vi "sensor test.vi"() -> ()   [LabVIEW 2019]
uses:
  <vilib>/vision/NI_Vision_Development_Module.lvlib
  defectsWrapper/defectsWrapper.lvlib
panel:
  out "sensor errors 2":errorcluster
  in  "stop 4":bool
  out "counter out":dbl
  out "defnum":dbl
  out "proc. ok":bool=TRUE
  out "x-y defects locs":dbl[][](array[numeric])
  in  "stop 3":bool
  out "crop array":dbl[][](array[numeric])
  out "Frm False":bool
  out "Pallet Defects View":T1(plugin-control)
  in  "size":dbl=5.0
  in  "threshoulds":dbl[](array[numeric])=[900.0, 1000.0, 1600.0, 2400.0, 3000.0, 3000.0]
  out "pallet detect":bool
  out "column count":bool
  out "error out 2":errorcluster
  in  "File Path":path=path "C:/Users/user/Pictures/saved pic"
  out "error out":errorcluster
  out "speed":dbl
  out "Image":T1(plugin-control)
  in  "stop 2":bool
  out "Image Out":T1(plugin-control)
  in  "Stop (F)":bool
  out "Waveform Chart 3":waveform(dbl)(graph)
  in  "Graph Button":bool
  out "capture or not?":bool=TRUE
  in  "capture":bool
  out "capture triger":bool
  in  "Color Box 4":u32(colorbox)=16448250
  in  "counting role":T2(ring)
  in  "timout":u32=50
  in  "Remote Port":u16=502
  out "IP #":string="169.254.116.245"
  in  "3rd sensor thr":u16=50000
  in  "2nd sensor thr":u16=52000
  in  "1st sensor thr":u32=52000
  in  "stop":bool
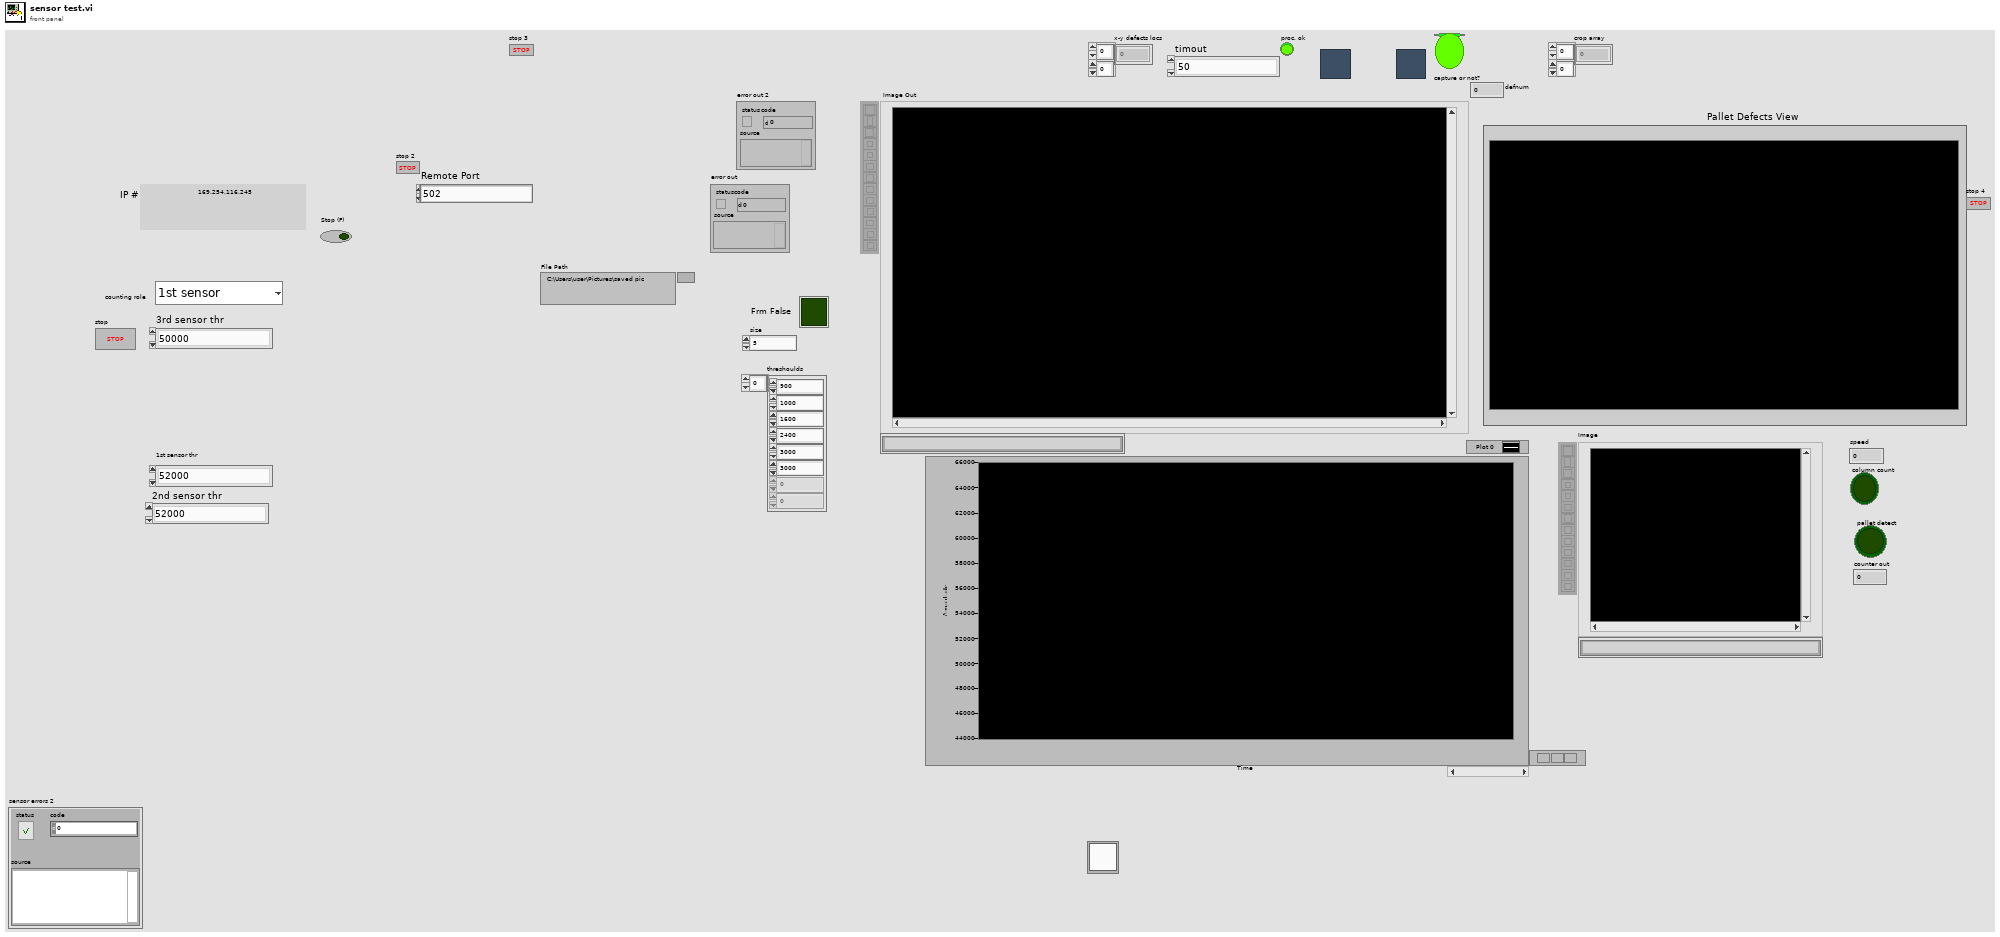
[diagram p1: front panel]
types:
  T1 = typedef "IMAQ Image.ctl" = refnum<image>
  T2 = enum16{"1st sensor", "2nd sensor", "3rd sensor", "1st+2nd", "1st+3rd", "2nd+3rd", "1st+2nd+3rd"}
  T3 = cluster{"ch sensor1":dbl, "ch sensor2":dbl, "ch sensor3":dbl, "ch sw sensor1":dbl, "ch sw sensor2":dbl}
  T4 = typedef "Image Type" = u32
  T5 = enum32{"Invalid", "Standard", "Closed", "Hidden", "Minimized", "Maximized"}
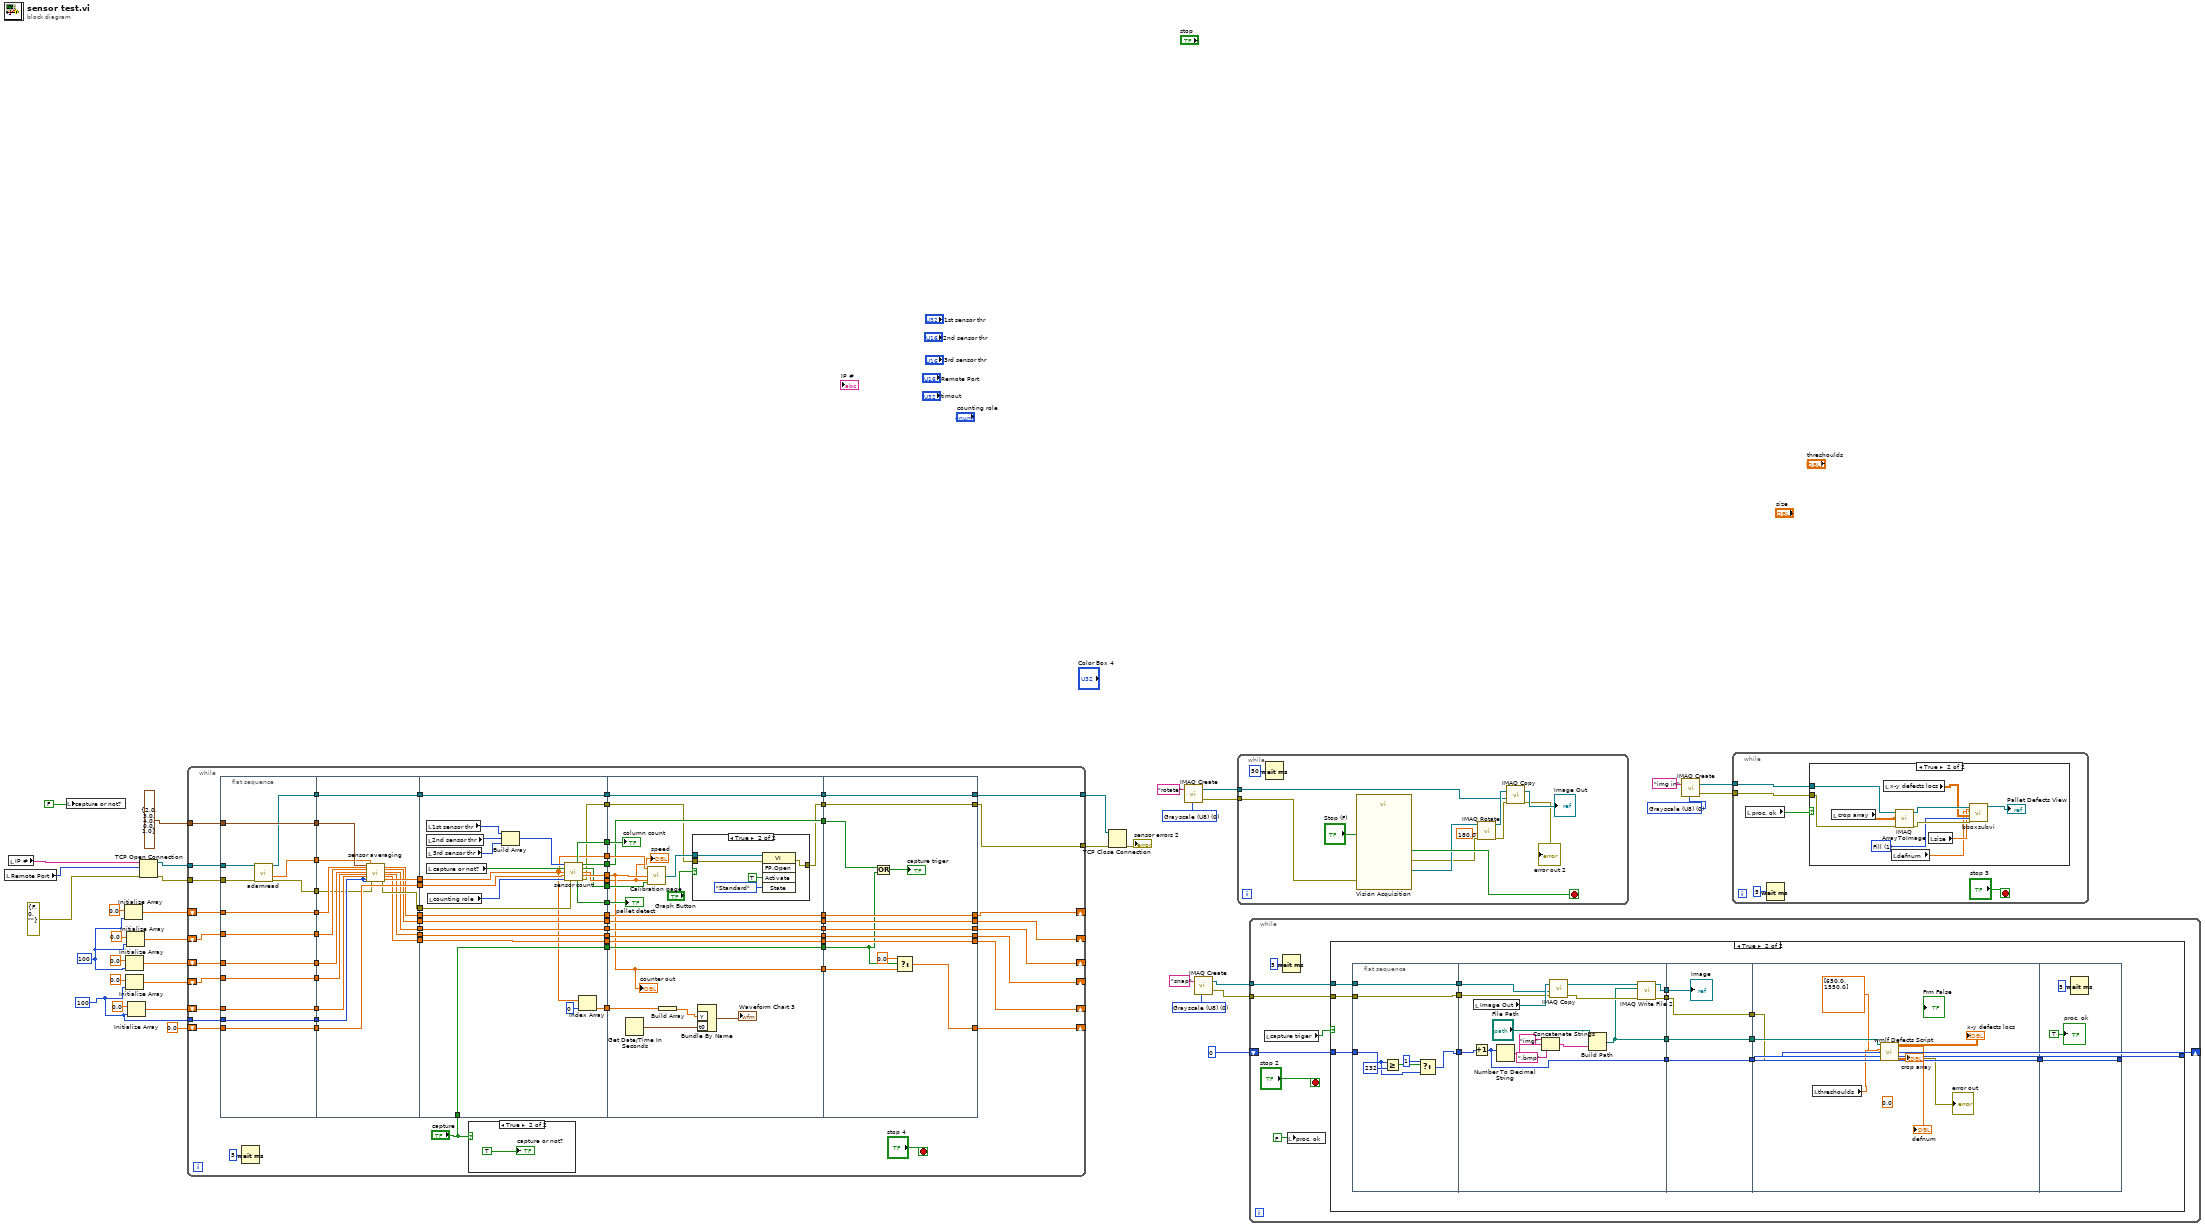
[diagram p0: block diagram]
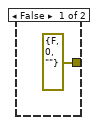
[diagram p3: hidden frame]
diagram:
  w5 = 100 ("dimension size")
  w15 = 100 ("dimension size")
  w25 = T4 0 items=["Grayscale (U8)", "Grayscale (I16)", "Grayscale (SGL)", "Complex (CSG)", "RGB (U32)", "HSL (U32)", "RGB (U64)", "Grayscale (U16)"] ("Image Type")
  w29 = T4 0 items=["Grayscale (U8)", "Grayscale (I16)", "Grayscale (SGL)", "Complex (CSG)", "RGB (U32)", "HSL (U32)", "RGB (U64)", "Grayscale (U16)"] ("Image Type")
  w36 = T4 0 items=["Grayscale (U8)", "Grayscale (I16)", "Grayscale (SGL)", "Complex (CSG)", "RGB (U32)", "HSL (U32)", "RGB (U64)", "Grayscale (U16)"] ("Image Type")
  n1 = local read "Remote Port"() -> (w21:u16)
  n2 = local read "IP #"() -> (w20:string)
  n3 = local write "capture or not?"(FALSE ("Boolean 2")) -> ()
  n4 = Initialize Array(0.0 ("element"), w15) -> (w11:dbl[])
  n5 = Initialize Array(0.0 ("element"), w15) -> (w9:dbl[])
  n6 = Initialize Array(0.0 ("element"), w5) -> (w8:dbl[])
  n7 = Initialize Array(0.0 ("element"), w15) -> (w10:dbl[])
  n8 = Initialize Array(0.0 ("element"), w5) -> (w7:dbl[])
  n9 = TCP Open Connection(address=w20, remote port or service name=w21, error in (no error)=errorcluster {"status"=FALSE, "code"=0, "source"=""}) -> (connection ID=w19:refnum<k5>, error out=w18:errorcluster)  [unwired: 2 in]
  n10 = while {
    tunnel: w19 -> [w103]
    tunnel: w18 -> [w102]
    shift-right: [w78] -> _
    shift-left: w11 -> [w97]
    shift-right: [w75] -> _
    shift-left: w10 -> [w95]
    shift-right: [w72] -> _
    shift-left: w9 -> [w93]
    shift-right: [w69] -> _
    shift-left: w8 -> [w91]
    shift-right: [w66] -> _
    shift-left: w7 -> [w90]
    tunnel: T3 {"ch sensor1"=2.0, "ch sensor2"=3.0, "ch sensor3"=4.0, "ch sw sensor1"=0.0, "ch sw sensor2"=1.0} ("cluster") -> [w99]
    tunnel: w5 -> [w87]
    shift-right: [w47] -> _
    shift-left: 0.0 ("element") -> [w48]
    tunnel: [w38] -> w3
    tunnel: [w37] -> w2
    stop <- "stop 4" stop-if-true
    n11 = flat-sequence {
      tunnel: w103 -> [w117]
      tunnel: w102 -> [w116]
      tunnel: [w115] -> w100
      tunnel: w99 -> [w115]
      tunnel: [w114] -> w98
      tunnel: w97 -> [w114]
      tunnel: [w113] -> w96
      tunnel: w95 -> [w113]
      tunnel: [w112] -> w94
      tunnel: w93 -> [w112]
      tunnel: [w111] -> w92
      tunnel: w91 -> [w111]
      tunnel: w90 -> [w110]
      tunnel: [w110] -> w89
      tunnel: [w109] -> w88
      tunnel: w87 -> [w109]
      tunnel: [w108] -> w86
      tunnel: w48 -> [w107]
      tunnel: [w107] -> w84
      tunnel: [w106] -> w82
      tunnel: [w105] -> w39
      tunnel: w100 -> [w135]
      tunnel: w98 -> [w134]
      tunnel: w96 -> [w133]
      tunnel: w94 -> [w132]
      tunnel: w92 -> [w131]
      tunnel: w89 -> [w130]
      tunnel: w88 -> [w129]
      tunnel: w86 -> [w128]
      tunnel: [w127] -> w85
      tunnel: w84 -> [w126]
      tunnel: [w126] -> w83
      tunnel: w82 -> [w125]
      tunnel: [w124] -> w81
      tunnel: [w123] -> w80
      tunnel: [w122] -> w77
      tunnel: [w121] -> w74
      tunnel: [w120] -> w70
      tunnel: [w119] -> w67
      tunnel: [w118] -> w40
      tunnel: w39 -> [w118]
      tunnel: w85 -> [w140]
      tunnel: w83 -> [w155]
      tunnel: w81 -> [w153]
      tunnel: w80 -> [w152]
      tunnel: [w152] -> w79
      tunnel: w77 -> [w151]
      tunnel: [w151] -> w76
      tunnel: w74 -> [w150]
      tunnel: [w150] -> w73
      tunnel: [w149] -> w71
      tunnel: w70 -> [w149]
      tunnel: [w148] -> w68
      tunnel: w67 -> [w148]
      tunnel: [w140] -> w65
      tunnel: [w147] -> w64
      tunnel: [w146] -> w63
      tunnel: [w145] -> w62
      tunnel: [w144] -> w61
      tunnel: [w143] -> w60
      tunnel: [w142] -> w53
      tunnel: "capture" -> [w142]
      tunnel: [w141] -> w50
      tunnel: [w138] -> w46
      tunnel: [w137] -> w43
      tunnel: [w136] -> w41
      tunnel: w40 -> [w136]
      tunnel: w79 -> [w182]
      tunnel: w76 -> [w181]
      tunnel: w73 -> [w180]
      tunnel: w71 -> [w179]
      tunnel: w68 -> [w178]
      tunnel: w65 -> [w177]
      tunnel: w64 -> [w169]
      tunnel: w63 -> [w168]
      tunnel: w62 -> [w176]
      tunnel: w61 -> [w175]
      tunnel: w60 -> [w174]
      tunnel: [w182] -> w59
      tunnel: [w181] -> w58
      tunnel: [w180] -> w57
      tunnel: [w179] -> w56
      tunnel: [w178] -> w55
      tunnel: [w171] -> w54
      tunnel: w53 -> [w171]
      tunnel: [w170] -> w51
      tunnel: w50 -> [w170]
      tunnel: [w169] -> w49
      tunnel: w46 -> [w166]
      tunnel: [w161] -> w44
      tunnel: w43 -> [w162]
      tunnel: [w163] -> w42
      tunnel: w41 -> [w163]
      tunnel: [w197] -> w66
      tunnel: [w198] -> w69
      tunnel: [w199] -> w72
      tunnel: [w200] -> w75
      tunnel: [w201] -> w78
      tunnel: w59 -> [w201]
      tunnel: w58 -> [w200]
      tunnel: w57 -> [w199]
      tunnel: w56 -> [w198]
      tunnel: w55 -> [w197]
      tunnel: w54 -> [w194]
      tunnel: w51 -> [w196]
      tunnel: w49 -> [w193]
      tunnel: [w191] -> w47
      tunnel: w44 -> [w190]
      tunnel: [w190] -> w38
      tunnel: [w189] -> w37
      tunnel: w42 -> [w189]
      frame #0 {
        n12 = call "adamread.vi"("TCP Connection Refnum in"=w117, "error in (no error)"=w116) -> ("TCP Connection Refnum (dup)"=w105:refnum<k5>, "Slave Input Registers 2"=w108:dbl[], "error out 2"=w106:errorcluster)  [unwired: 11 in]
      }
      frame #1 {
        n13 = call "sensor averaging.vi"("sensor chanel cluster"=w135, "array"=w134, "array 2"=w133, "array 3"=w132, "array 4"=w131, "array 5"=w130, "avg win1"=w129, "avg win2"=w129, "array sensor in"=w128, "error in"=w125) -> ("error out"=w124:errorcluster, "output array"=w123:dbl[], "output array 2"=w122:dbl[], "output array 3"=w121:dbl[], "output array 4"=w120:dbl[], "output array 5"=w119:dbl[], "avg data array"=w127:dbl[])  [unwired: 10 in, 1 out]
      }
      frame #2 {
        n14 = local read "1st sensor thr"() -> (w159:u32)
        n15 = local read "2nd sensor thr"() -> (w158:u16)
        n16 = local read "3rd sensor thr"() -> (w157:u16)
        n17 = local read "capture or not?"() -> (w160:bool)
        n18 = local read "counting role"() -> (w154:T2)
        n19 = Build Array(w159, w158, w157) -> (w156:u32[])
        n20 = call "sensor count.vi"("sensor thr array"=w156, "capture y or no ?"=w160, "sensor data"=w140, "counter input"=w155, "counting role"=w154, "error in"=w153) -> ("column count"=w144:bool, "capture trigger"=w141:bool, "sensor counter"=w145:bool, "speed"=w146:dbl, "counter out"=w147:dbl, "pallet detect"=w143:bool, "error out"=w137:errorcluster)  [unwired: 3 in]
        n21 = Index Array(array=w140, index=0) -> (element=w138:dbl)
      }
      frame #3 {
        n22 = Get Date/Time In Seconds() -> (seconds since 1Jan1904=w167:timestamp)
        n23 = call "Calibration page.vi"("sensor data array"=w177, "Numeric"=w169, "Speed (m/min) 2"=w168, "sensor count"=w176) -> ("This VI"=w173:refnum<vi>)  [unwired: 11 in]
        n24 = Build Array(w166) -> (w165:dbl[])
        n25 = case shown="True" "Graph Button" {
          tunnel: [errorcluster {"status"=FALSE, "code"=0, "source"=""} ("error out") w186] -> w161
          tunnel: w173 -> [_ w185]
          tunnel: w162 -> [_ w184]
          frame False {
          }
          frame True {
            n26 = invoke class="VI" method="FP.Open"(reference=w185, error in=w184, "Activate"=TRUE ("Activate?"), "State"=T5."Standard") -> (error out=w186:errorcluster)  [unwired: 1 in, 4 out]
          }
        }
        n27 = Bundle By Name("Y"=w165, "t0"=w167) -> (→"Waveform Chart 3":waveform(dbl))  [unwired: 1 in]
        "column count" <- w175
        "pallet detect" <- w174
        "counter out" <- w169
        "speed" <- w168
      }
      frame #4 {
        n28 = Or(x=w196, y=w194) -> (x .or. y?=→"capture triger":bool)
        n29 = Select(t=0.0, s=w194, f=w193) -> (s? t:f=w191:dbl)
      }
    }
    n30 = Wait (ms)(milliseconds to wait=u32 5) -> ()  [unwired: 1 out]
    n31 = case shown="True" "capture" {
      frame False {
      }
      frame True {
        "capture or not?" <- TRUE ("Boolean")
      }
    }
  }
  n32 = TCP Close Connection(connection ID=w2, error in (no error)=w3) -> (error out=→"sensor errors 2":errorcluster)  [unwired: 1 in, 1 out]
  n33 = call "IMAQ Create"("Image Name"="rotate", "Image Type"=w29) -> ("New Image"=w28:T1, "error out"=w27:errorcluster)  [unwired: 3 in]
  n34 = call "IMAQ Create"("Image Name"="snap", "Image Type"=w36) -> ("New Image"=w33:T1, "error out"=w32:errorcluster)  [unwired: 3 in]
  n35 = while {
    tunnel: w28 -> [w207]
    tunnel: w27 -> [w205]
    stop <- w212 stop-if-true
    n36 = Wait (ms)(milliseconds to wait=u32 50) -> ()  [unwired: 1 out]
    n37 = call "Vision Acquisition"("Stop (F)"="Stop (F)", "error in"=w205) -> ("Image Out"=w211:T1, "Stopped"=w212:bool, "error out"=w204:errorcluster)  [unwired: 23 in]
    n38 = call "IMAQ Rotate"("error in (no error)"=w204, "Angle (degrees)"=sgl 180.0, "Image Src"=w211) -> ("error out"=w203:errorcluster, "Image Dst Out"=w208:T1)  [unwired: 7 in]
    n39 = call "IMAQ Copy"("error in (no error)"=w203, "Image Dst"=w207, "Image Src"=w208) -> ("error out"=→"error out 2":errorcluster, "Image Dst Out"=→"Image Out":T1)  [unwired: 3 in]
  }
  n40 = while {
    tunnel: w33 -> [w219]
    tunnel: w32 -> [w218]
    shift-right: [w215] -> _
    shift-left: 0 -> [w216]
    stop <- "stop 2" stop-if-true
    n41 = local read "capture triger"() -> (w220:bool)
    n42 = Wait (ms)(milliseconds to wait=u32 5) -> ()  [unwired: 1 out]
    n43 = local write "proc. ok"(FALSE ("proc. ok")) -> ()
    n44 = case shown="True" w220 {
      tunnel: w219 -> [_ w237]
      tunnel: w218 -> [_ w234]
      tunnel: w216 -> [w222 w230]
      tunnel: [w222 w229] -> w215
      frame False {
      }
      frame True {
        n45 = flat-sequence {
          tunnel: w237 -> [w244]
          tunnel: [w244] -> w236
          tunnel: [w243] -> w235
          tunnel: w234 -> [w243]
          tunnel: [w238] -> w231
          tunnel: w230 -> [w239]
          tunnel: w236 -> [w257]
          tunnel: w235 -> [w258]
          tunnel: [w254] -> w233
          tunnel: [w253] -> w232
          tunnel: w231 -> [w250]
          tunnel: [w246] -> w228
          tunnel: [w245] -> w226
          tunnel: w233 -> [w263]
          tunnel: w232 -> [w260]
          tunnel: w228 -> [w262]
          tunnel: [w262] -> w227
          tunnel: w226 -> [w261]
          tunnel: [w261] -> w225
          tunnel: [w260] -> w224
          tunnel: w227 -> [w272]
          tunnel: w225 -> [w271]
          tunnel: w224 -> [w270]
          tunnel: [w272] -> w223
          tunnel: [w275] -> w229
          tunnel: w223 -> [w275]
          frame #0 {
            n46 = Greater Or Equal?(x=w239, y=232) -> (x >= y?=w241:bool)
            n47 = Select(t=i8 1, s=w241, f=w239) -> (s? t:f=w238:i32)
          }
          frame #1 {
            n48 = Increment(x=w250) -> (x+1=w246:i32)
            n49 = local read "Image Out"() -> (w259:T1)
            n50 = Number To Decimal String(number=w246) -> (decimal integer string=w249:string)  [unwired: 1 in]
            n51 = Concatenate Strings("img" ("string"), w249, ".bmp" ("string")) -> (w247:string)
            n52 = call "IMAQ Copy"("error in (no error)"=w258, "Image Dst"=w257, "Image Src"=w259) -> ("error out"=w255:errorcluster, "Image Dst Out"=w256:T1)  [unwired: 3 in]
            n53 = Build Path(base path="File Path", name or relative path=w247) -> (appended path=w245:path)
            n54 = call-poly "IMAQ Write File 2"("error in (no error)"=w255, "File Path"=w245, "Image"=w256) -> ("error out"=w253:errorcluster, "Image Out (duplicate)"=w254:T1)  [unwired: 7 in]
          }
          frame #2 {
            "Image" <- w263
          }
          frame #3 {
            (unwired) 0.0 ("defect ratio 2")
            n55 = local read "threshoulds"() -> (w269:dbl[])
            n56 = call "wmlf Defects Script.vi"("File Path"=w271, "threshoulds"=w269, "margin"=dbl[] [650.0, 1550.0], "error in (no error)"=w270) -> ("x-y defects locs"=→"x-y defects locs":dbl[][], "defnum"=→"defnum":dbl, "crop array"=→"crop array":dbl[][], "error out"=→"error out":errorcluster)  [unwired: 16 in, 4 out]
          }
          frame #4 {
            n57 = Wait (ms)(milliseconds to wait=u32 5) -> ()  [unwired: 1 out]
            "proc. ok" <- TRUE
          }
        }
      }
    }
  }
  n58 = call "IMAQ Create"("Image Name"="img in", "Image Type"=w25) -> ("New Image"=w24:T1, "error out"=w23:errorcluster)  [unwired: 3 in]
  n59 = while {
    tunnel: w24 -> [w279]
    tunnel: w23 -> [w278]
    stop <- "stop 3" stop-if-true
    n60 = local read "proc. ok"() -> (w276:bool)
    n61 = Wait (ms)(milliseconds to wait=u32 5) -> ()  [unwired: 1 out]
    n62 = case shown="True" w276 {
      tunnel: w279 -> [_ w289]
      tunnel: w278 -> [_ w288]
      frame False {
      }
      frame True {
        w284 = u32 1 items=["Frame", "Fill"] ("Drawing Mode (Frame)")
        n63 = local read "crop array"() -> (w290:dbl[][])
        n64 = local read "x-y defects locs"() -> (w286:dbl[][])
        n65 = local read "defnum"() -> (w282:dbl)
        n66 = call "IMAQ ArrayToImage"("error in (no error)"=w288, "Image Pixels (U8)"=w290, "Image"=w289) -> ("error out"=w285:errorcluster, "Image Out"=w287:T1)  [unwired: 7 in]
        n67 = local read "size"() -> (w283:dbl)
        n68 = call "bboxsubvi.vi"("Image"=w287, "size"=w283, "def num"=w282, "array"=w286, "Drawing Mode (Frame)"=w284, "error in"=w285) -> ("Image Out"=→"Pallet Defects View":T1)  [unwired: 12 in, 1 out]
      }
    }
  }
